vi "Read Search.vi"(11 "Dependency in":refnum<class "Dependency.lvclass">) -> (2 "Search":refnum<class "Search.lvclass">, 3 "Dependency out":refnum<class "Dependency.lvclass">)   [LabVIEW 2016, in "Dependency.lvclass"]
uses:
  Dependency.lvclass
  Search/Search.lvclass
  Dependency.lvclass/Dependency.ctl
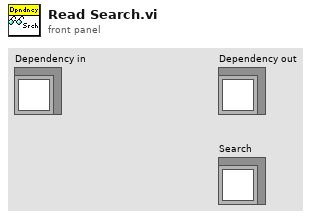
[diagram p1: front panel]
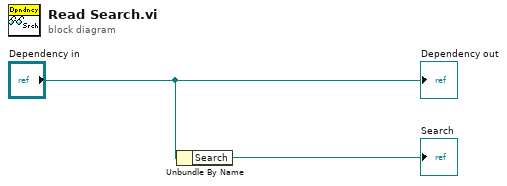
[diagram p0: block diagram]
diagram:
  n1 = Unbundle By Name("Dependency in") -> ("Search"=→"Search":refnum<class "Search.lvclass">)
  "Dependency out" <- "Dependency in"
